vi "removeDuplicates.vi"(8 "error in (no error)":errorcluster, 10 "times":dbl[](array[numeric]), 11 "RfOutputData in":refnum<class "RfOutputData.lvclass">) -> (0 "error out":errorcluster, 2 "times out":dbl[](array[numeric]), 3 "RfOutputData out":refnum<class "RfOutputData.lvclass">)   [LabVIEW 2009, in "DataMappers.lvlib" / "RfOutputData.lvclass"]
uses:
  RfOutputData.lvclass
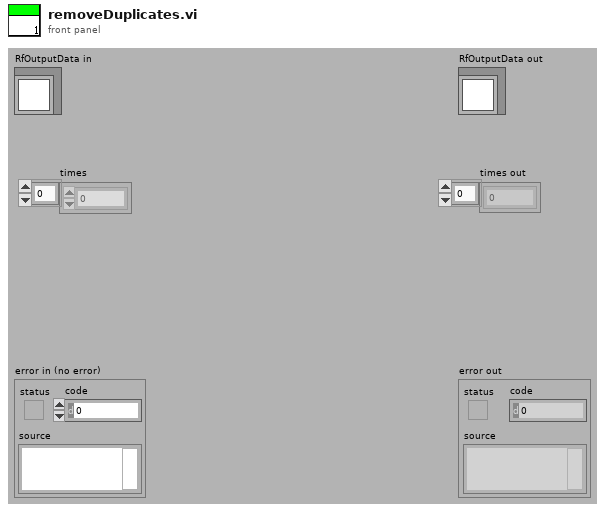
[diagram p1: front panel]
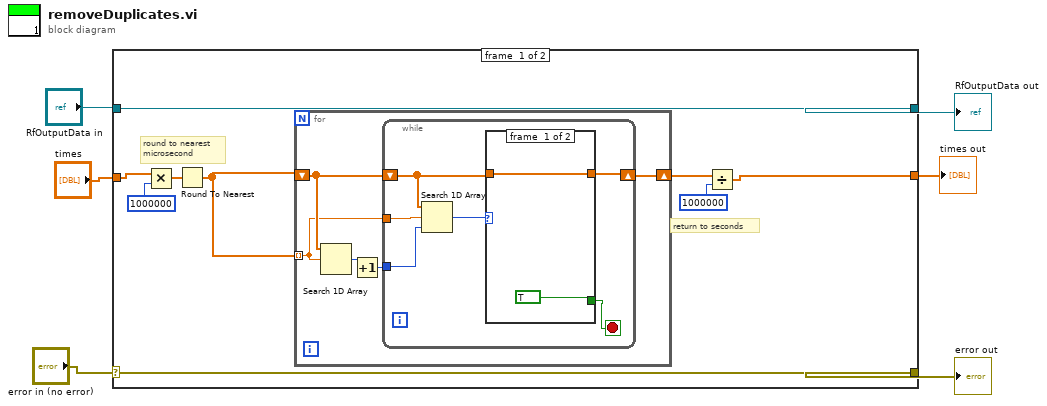
[diagram p0: block diagram]
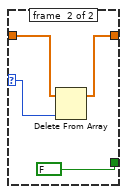
[diagram p2: hidden frame]
diagram:
  n1 = case shown="No Error" "error in (no error)" {
    selector: "error in (no error)" -> [w15 w35]
    tunnel: [w15 w35] -> w3
    tunnel: [w9 w34] -> w6
    tunnel: [w7 w33] -> w1
    tunnel: "RfOutputData in" -> [w9 w34]
    tunnel: "times" -> [w8 w33]
    frame #0 {
      # "return to seconds"
      # "round to nearest\nmicrosecond"
      n2 = Multiply(x=w8, y=1000000) -> (x*y=w13:dbl[])
      n3 = Round To Nearest(number=w13) -> (nearest integer value=w12:dbl[])
      n4 = for {
        shift-right: [w20] -> w11
        shift-left: w12 -> [w17]
        tunnel: w12 -> [w16] mode=indexing
        n5 = Search 1D Array(1D array=w17, element=w16) -> (index of element=w19:i32)  [unwired: 1 in]
        n6 = Increment(x=w19) -> (x+1=w18:i32)
        n7 = while {
          shift-right: [w24] -> w20
          shift-left: w17 -> [w22]
          tunnel: w18 -> [w23]
          tunnel: w16 -> [w21]
          stop <- w25 stop-if-true
          n8 = Search 1D Array(1D array=w22, element=w21, start index (0)=w23) -> (index of element=w26:i32)
          n9 = case shown="-1" w26 {
            selector: w26 -> [_ w31]
            tunnel: [TRUE FALSE] -> w25
            tunnel: w22 -> [w27 w30]
            tunnel: [w27 w29] -> w24
            frame #0 {
            }
            frame #1 {
              n10 = Delete From Array(array=w30, index=w31) -> (array with subset deleted=w29:dbl[])  [unwired: 1 in, 1 out]
            }
          }
        }
      }
      n11 = Divide(x=w11, y=1000000) -> (x/y=w7:dbl[])
    }
    frame #1 {
    }
  }
  "error out" <- w3
  "RfOutputData out" <- w6
  "times out" <- w1
